vi "Verity_SW1-5.vi"(8 "error in":errorcluster, 9 "Output Switch ID":i32, 10 "Input Switch ID":i32, 11 "Base Switch ID":i32) -> (0 "error out":errorcluster, 3 "Verfied":bool)   [LabVIEW 2012]
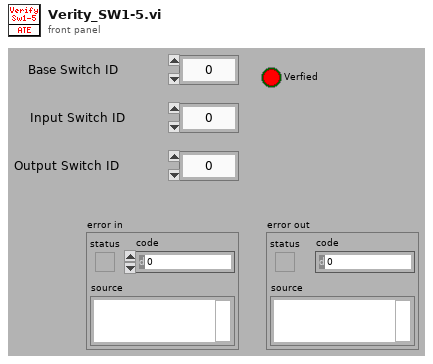
[diagram p1: front panel]
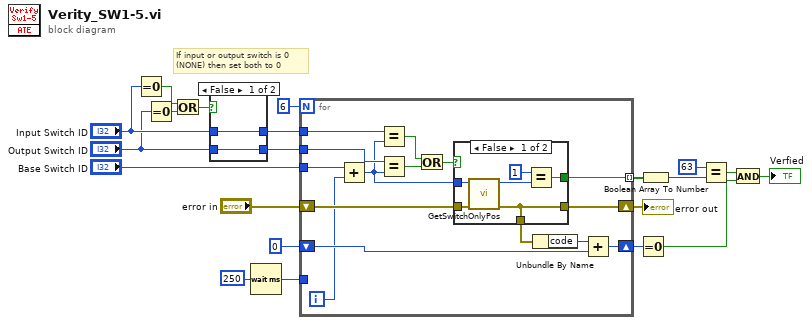
[diagram p0: block diagram]
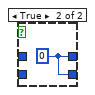
[diagram p2: hidden frame]
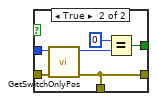
[diagram p3: hidden frame]
diagram:
  # "If input or output switch is 0\n(NONE) then set both to 0"
  n1 = Equal To 0?(x="Input Switch ID") -> (x = 0?=w8:bool)
  n2 = Equal To 0?(x="Output Switch ID") -> (x = 0?=w7:bool)
  n3 = Or(x=w8, y=w7) -> (x .or. y?=w4:bool)
  n4 = case shown="False" w4 {
    tunnel: "Input Switch ID" -> [w23 _]
    tunnel: "Output Switch ID" -> [w22 _]
    tunnel: [w23 w24] -> w3
    tunnel: [w22 w24] -> w2
    frame False {
    }
    frame True {
      w24 = 0 ("Input Switch ID")
    }
  }
  n5 = Wait (ms)(milliseconds to wait=u32 250) -> (millisecond timer value=w10:u32)
  n6 = for {
    N: 6 -> [_]
    tunnel: "Base Switch ID" -> [w39]
    tunnel: w3 -> [w38]
    tunnel: w2 -> [w37]
    tunnel: [w32] -> w19 mode=indexing
    shift-right: [w29] -> w15
    shift-left: 0 -> [w30]
    tunnel: w10 -> [_]
    shift-right: [w25] -> w1
    shift-left: "error in" -> [w33]
    i -> [w28]
    n7 = Add(x=w39, y=w28) -> (x+y=w31:i32)
    n8 = Equal?(x=w38, y=w31) -> (x = y?=w36:bool)
    n9 = Equal?(x=w37, y=w31) -> (x = y?=w35:bool)
    n10 = Or(x=w36, y=w35) -> (x .or. y?=w34:bool)
    n11 = case shown="False" w34 {
      tunnel: [w41 w49] -> w32
      tunnel: w31 -> [w43 w48]
      tunnel: w33 -> [w42 w47]
      tunnel: [w40 w46] -> w27
      tunnel: [w40 w46] -> w25
      frame False {
        n12 = call "GetSwitchOnlyPos.vi"("error in (no error)"=w42, "Circuit ID"=w43) -> ("Error out"=w40:errorcluster, "Position (0=open, 1=closed)"=w44:i32)  [unwired: 4 in]
        n13 = Equal?(x=1 ("Position (0=open, 1=closed)"), y=w44) -> (x = y?=w41:bool)
      }
      frame True {
        n14 = call "GetSwitchOnlyPos.vi"("error in (no error)"=w47, "Circuit ID"=w48) -> ("Error out"=w46:errorcluster, "Position (0=open, 1=closed)"=w51:i32)  [unwired: 4 in]
        n15 = Equal?(x=0 ("Position (0=open, 1=closed)"), y=w51) -> (x = y?=w49:bool)
      }
    }
    n16 = Unbundle By Name(w27) -> ("code"=w26:i32)
    n17 = Add(x=w26, y=w30) -> (x+y=w29:i32)
  }
  "error out" <- w1
  n18 = Equal To 0?(x=w15) -> (x = 0?=w13:bool)
  n19 = Boolean Array To Number(Boolean array=w19) -> (number=w18:u32)
  n20 = Equal?(x=u32 63, y=w18) -> (x = y?=w14:bool)
  n21 = And(x=w14, y=w13) -> (x .and. y?=→"Verfied":bool)
